vi "getState.vi"(8 "error in (no error)":errorcluster, 10 "dofIdx":i16[](array[numeric]), 11 "OptCtrl in":refnum<class "OptCtrl.lvclass">) -> (0 "error out":errorcluster, 2 "State in DOF":dbl[](array[numeric]), 3 "OptCtrl out":refnum<class "OptCtrl.lvclass">)   [LabVIEW 2016, in "OptCtrl.lvclass"]
doc: "Get the state (x) in degree of freedom (DOF)."
uses:
  OptCtrl.lvclass
  OptCtrl.lvclass/OptCtrl.ctl
  Utility/getSubArray1D.vi
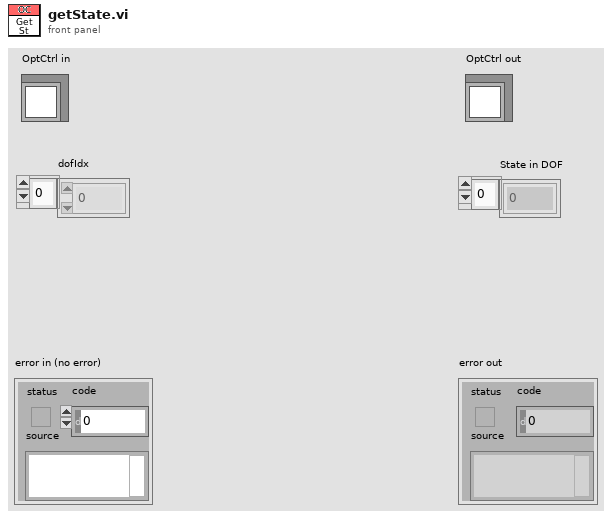
[diagram p1: front panel]
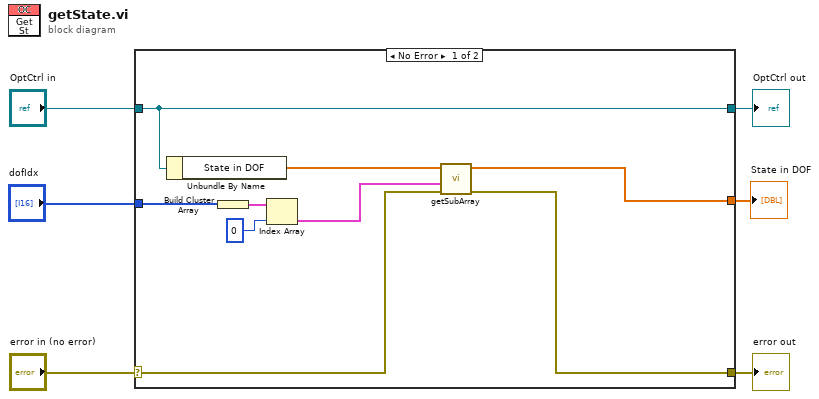
[diagram p0: block diagram]
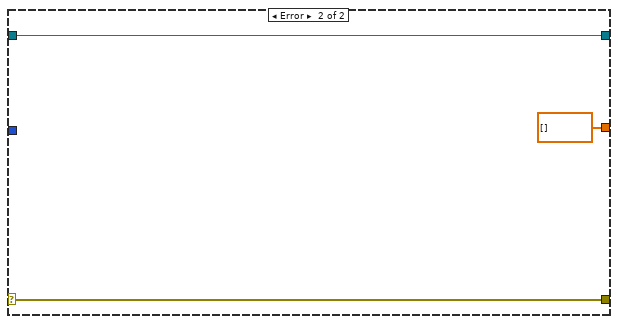
[diagram p2: hidden frame]
diagram:
  n1 = case shown="No Error" "error in (no error)" {
    selector: "error in (no error)" -> [w9 w18]
    tunnel: [w8 w18] -> w5
    tunnel: [w15 w17] -> w3
    tunnel: "OptCtrl in" -> [w15 w17]
    tunnel: [w7 dbl[] [] ("State in DOF")] -> w2
    tunnel: "dofIdx" -> [w11 _]
    frame No Error {
      n2 = Unbundle By Name(w15) -> ("State in DOF"=w12:dbl[])
      n3 = Build Cluster Array(w11) -> (w14:cluster{"dofIdx":i16[]}[])
      n4 = Index Array(array=w14, index=0) -> (element=w10:cluster{"dofIdx":i16[]})
      n5 = call-poly "getSubArray.vi"("error in (no error)"=w9, "Index Array Cluster"=w10, "1D Array"=w12) -> ("error out"=w8:errorcluster, "Sub-Array"=w7:dbl[])  [unwired: 7 in]
    }
    frame Error {
    }
  }
  "error out" <- w5
  "OptCtrl out" <- w3
  "State in DOF" <- w2
